vi "Table Manager.vi"(6 "Entry ID in":T1, 8 "Operation":T2, 10 "Entry Name":string) -> (0 "Entries":cluster{"Entry IDs":T1[], "Names":string[]}, 1 "Success":bool, 2 "Entry ID":T1, 4 "Entry Name":string)   [LabVIEW 2017]
doc: "Manges the Name to Entry ID map. Can be used to lookup an entry's ID, add, delete, etc."
uses:
  <vilib>/Rock Robotics/Network Tables/Field ID.ctl
  <vilib>/Rock Robotics/Network Tables/Make Table Operation.ctl
  <vilib>/Rock Robotics/Network Tables/NT Globals.vi
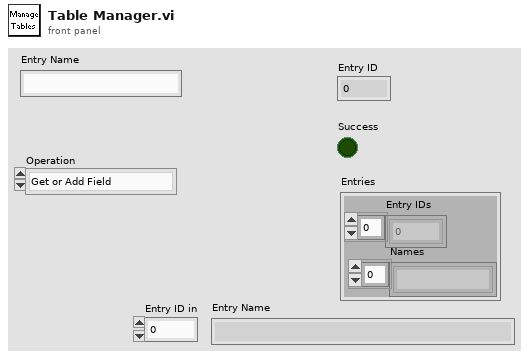
[diagram p1: front panel]
types:
  T1 = typedef "Field ID.ctl" = i32
  T2 = typedef "Make Table Operation.ctl" = enum16{"Get or Add Field", "Get Field or Add Temp", "Replace Temp ID", "Get Field ID - No Add", "Get Table Field IDs", "Get Field ID Info", "Move Field to Temp", "Validate", "Remove Field", "Remove All"}
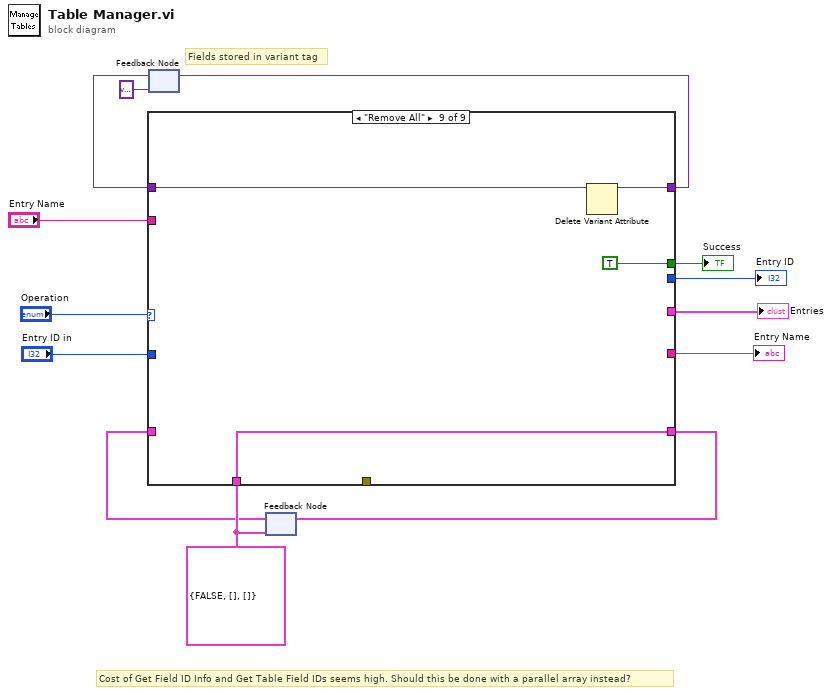
[diagram p0: block diagram]
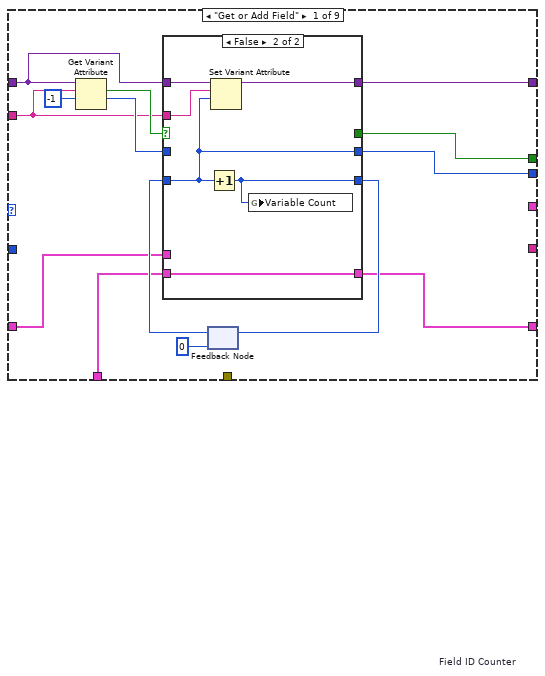
[diagram p2: hidden frame]
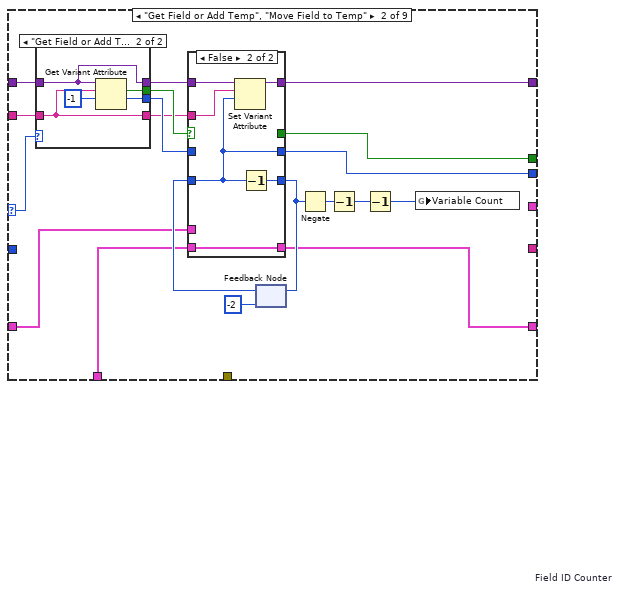
[diagram p4: hidden frame]
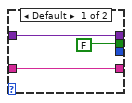
[diagram p5: hidden frame]
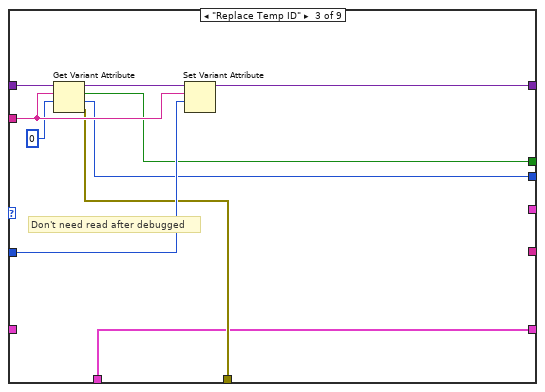
[diagram p7: hidden frame]
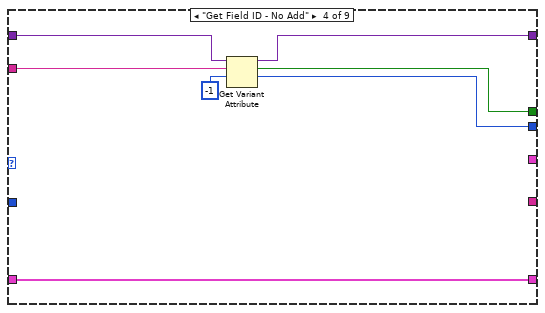
[diagram p8: hidden frame]
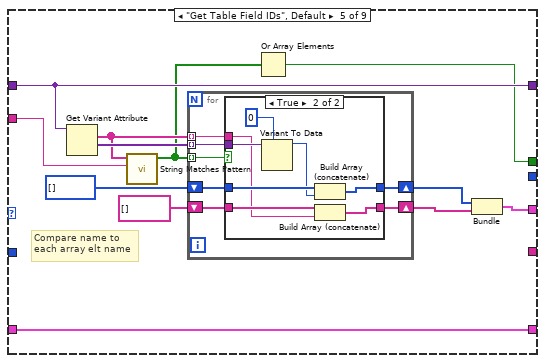
[diagram p9: hidden frame]
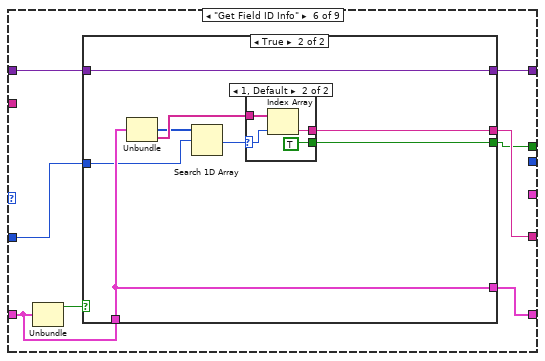
[diagram p11: hidden frame]
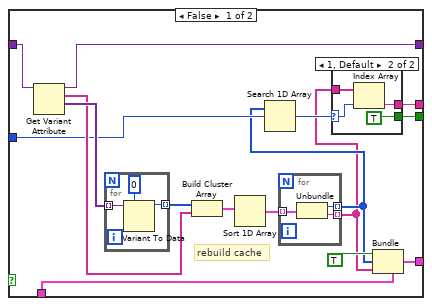
[diagram p12: hidden frame]
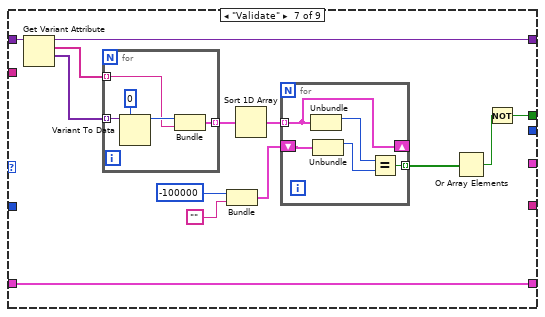
[diagram p15: hidden frame]
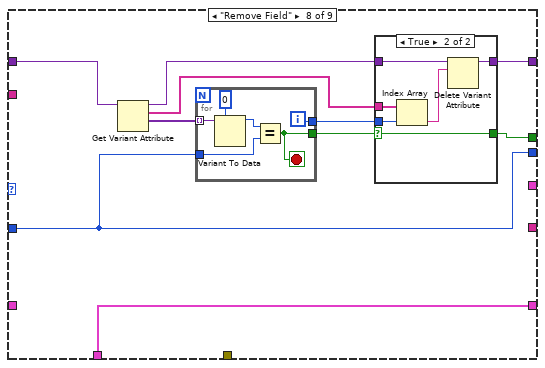
[diagram p16: hidden frame]
diagram:
  w3 = cluster{bool, i32[], string[]} {FALSE, [], []}
  # "Cost of Get Field ID Info and Get Table Field IDs seems high. Should this be done with a parallel array instead?"
  # "Fields stored in variant tag"
  n1 = feedback #1(variant ("Variant")) -> (w7:variant)
  n2 = feedback #2(w3) -> (w2:cluster{bool, i32[], string[]})
  n3 = case shown="\"Remove All\"" "Operation" {
    selector: "Operation" -> [_ w48 _ _ _ _ _ _ _]
    tunnel: w7 -> [w17 w50 w86 w89 w105 w127 w181 w197 w217]
    tunnel: [w21 w51 w81 w88 w105 w126 w180 w194 w219] -> w8
    tunnel: [w25 w55 w82 w91 w95 w124 w171 w196 TRUE] -> w12
    tunnel: "Entry Name" -> [w20 w47 w84 w93 w98 _ _ _ _]
    tunnel: [w26 w56 w79 w92 _ _ _ w193 _] -> w10
    tunnel: "Entry ID in" -> [_ _ w83 _ _ w130 _ w193 _]
    tunnel: [_ _ _ _ _ w125 _ _ _] -> w6
    tunnel: [_ _ _ _ w101 _ _ _ _] -> w4
    tunnel: [_ _ w78 _ _ _ _ _ _] -> _
    tunnel: w3 -> [w15 w40 w77 _ _ _ _ w192 w216]
    tunnel: w2 -> [w16 w41 _ w87 w94 w128 w169 _ _]
    tunnel: [w14 w39 w77 w87 w94 w123 w169 w192 w216] -> w1
    frame "Get or Add Field" {
      n4 = Get Variant Attribute(Variant=w17, name=w20, default value (empty Variant)=-1) -> (found=w24:bool, value=w23:i32)  [unwired: 1 in, 2 out]
      n5 = feedback #3 "Field ID Counter"(0) -> (w19:i32)
      n6 = case shown="False" w24 {
        selector: w24 -> [w30 _]
        tunnel: w17 -> [w32 w37]
        tunnel: [w32 w36] -> w21
        tunnel: w20 -> [_ w38]
        tunnel: [w30 _] -> w25
        tunnel: w19 -> [w29 w35]
        tunnel: [w31 w35] -> w26
        tunnel: w23 -> [w31 _]
        tunnel: [w29 w34] -> w18
        tunnel: w16 -> [w28 _]
        tunnel: w15 -> [_ w33]
        tunnel: [w28 w33] -> w14
        frame True {
          # "Already present"
        }
        frame False {
          n7 = Increment(x=w35) -> (x+1=w34:i32)
          n8 = Set Variant Attribute(Variant=w37, name=w38, value=w35) -> (Variant out=w36:variant)  [unwired: 1 in, 2 out]
          n9 = global write "NT Globals.vi" "Variable Count"(w34) -> ()
        }
      }
      n10 = feedback-in #3(w18) -> ()
    }
    frame "Get Field or Add Temp", "Move Field to Temp" {
      n11 = case shown="\"Get Field or Add Temp\"" w48 {
        tunnel: [FALSE ("Autonomous") w65] -> w54
        tunnel: [_ w64] -> w53
        tunnel: [w59 w61] -> w52
        tunnel: w50 -> [w59 w61]
        tunnel: w47 -> [w60 w63]
        tunnel: [w60 w63] -> w46
        frame Default {
        }
        frame "Get Field or Add Temp" {
          n12 = Get Variant Attribute(Variant=w61, name=w63, default value (empty Variant)=-1) -> (found=w65:bool, value=w64:i32)  [unwired: 1 in, 2 out]
        }
      }
      n13 = feedback #4 "Field ID Counter"(-2) -> (w49:i32)
      n14 = case shown="False" w54 {
        selector: w54 -> [w68 _]
        tunnel: w52 -> [w70 w75]
        tunnel: [w70 w74] -> w51
        tunnel: w46 -> [_ w76]
        tunnel: [w68 _] -> w55
        tunnel: w49 -> [w67 w73]
        tunnel: [w69 w73] -> w56
        tunnel: w53 -> [w69 _]
        tunnel: [w67 w72] -> w45
        tunnel: w41 -> [w66 _]
        tunnel: w40 -> [_ w71]
        tunnel: [w66 w71] -> w39
        frame True {
          # "Already\npresent"
        }
        frame False {
          n15 = Set Variant Attribute(Variant=w75, name=w76, value=w73) -> (Variant out=w74:variant)  [unwired: 1 in, 2 out]
          n16 = Decrement(x=w73) -> (x-1=w72:i32)
        }
      }
      n17 = feedback-in #4(w45) -> ()
      n18 = Negate(x=w45) -> (-x=w44:i32)
      n19 = Decrement(x=w44) -> (x-1=w43:i32)
      n20 = Decrement(x=w43) -> (x-1=w42:i32)
      n21 = global write "NT Globals.vi" "Variable Count"(w42) -> ()
    }
    frame "Replace Temp ID" {
      # "Don't need read after debugged"
      n22 = Get Variant Attribute(Variant=w86, name=w84, default value (empty Variant)=T1 0 ("Entry ID")) -> (duplicate Variant=w85:variant, found=w82:bool, value=w79:T1, error out=w78:errorcluster)  [unwired: 1 in]
      n23 = Set Variant Attribute(Variant=w85, name=w84, value=w83) -> (Variant out=w81:variant)  [unwired: 1 in, 2 out]
    }
    frame "Get Field ID - No Add" {
      n24 = Get Variant Attribute(Variant=w89, name=w93, default value (empty Variant)=-1) -> (duplicate Variant=w88:variant, found=w91:bool, value=w92:i32)  [unwired: 1 in, 1 out]
    }
    frame "Get Table Field IDs", Default {
      # "Compare name to\neach array elt name"
      n25 = Get Variant Attribute(Variant=w105) -> (names=w97:string[], values=w104:variant[])  [unwired: 3 in, 2 out]
      n26 = call <vilib>:"String Matches Pattern.vi"("Pattern"=w98, "Names"=w97) -> ("Matching"=w96:bool[])  [unwired: 9 in]
      n27 = for {
        tunnel: w104 -> [w112] mode=indexing
        tunnel: w97 -> [w107] mode=indexing
        shift-right: [w109] -> w102
        shift-left: i32[] [] -> [w111]
        shift-right: [w108] -> w103
        shift-left: string[] [] ("names") -> [w110]
        tunnel: w96 -> [w106] mode=indexing
        n28 = case shown="True" w106 {
          tunnel: w112 -> [_ w122]
          tunnel: w111 -> [w114 w118]
          tunnel: w110 -> [w113 w120]
          tunnel: [w114 w117] -> w109
          tunnel: [w113 w119] -> w108
          tunnel: w107 -> [_ w115]
          frame False {
          }
          frame True {
            n29 = Variant To Data(type=0, Variant=w122) -> (data=w116:i32)  [unwired: 1 in, 1 out]
            n30 = Build Array (concatenate)(w118, w116) -> (w117:i32[])
            n31 = Build Array (concatenate)(w120, w115) -> (w119:string[])
          }
        }
      }
      n32 = Or Array Elements(Boolean array=w96) -> (logical OR=w95:bool)
      n33 = Bundle(w102, "names"=w103) -> (w101:cluster{i32[], "names":string[]})  [unwired: 1 in]
    }
    frame "Get Field ID Info" {
      n34 = Unbundle(w128) -> (w129:bool)  [unwired: 2 out]
      n35 = case shown="True" w129 {
        tunnel: w130 -> [w134 w159]
        tunnel: [w146 w162] -> w125
        tunnel: w127 -> [w145 w161]
        tunnel: [w144 w161] -> w126
        tunnel: [w143 w163] -> w124
        tunnel: [w141 w160] -> w123
        tunnel: w128 -> [w140 w160]
        frame False {
          # "rebuild cache"
          n36 = Get Variant Attribute(Variant=w145) -> (duplicate Variant=w144:variant, names=w137:string[], values=w139:variant[])  [unwired: 3 in, 1 out]
          n37 = for {
            tunnel: w139 -> [w152] mode=indexing
            tunnel: [w150] -> w138 mode=indexing
            n38 = Variant To Data(type=0, Variant=w152) -> (data=w150:i32)  [unwired: 1 in, 1 out]
          }
          n39 = Build Cluster Array(w138, w137) -> (w136:cluster{i32, string}[])
          n40 = Sort 1D Array(array=w136) -> (sorted array=w135:cluster{i32, string}[])
          n41 = for {
            tunnel: w135 -> [w149] mode=indexing
            tunnel: [w148] -> w133 mode=indexing
            tunnel: [w147] -> w131 mode=indexing
            n42 = Unbundle(w149) -> (w148:i32, w147:string)
          }
          n43 = Search 1D Array(1D array=w133, element=w134) -> (index of element=w132:i32)  [unwired: 1 in]
          n44 = case shown="1, Default" w132 {
            selector: w132 -> [_ w154]
            tunnel: w131 -> [_ w156]
            tunnel: [_ w155] -> w146
            tunnel: [_ TRUE] -> w143
            frame -1 {
            }
            frame 1, Default {
              n45 = Index Array(array=w156, index=w154) -> (element=w155:string)
            }
          }
          n46 = Bundle(cluster=w140, TRUE, w133, w131) -> (w141:cluster{bool, i32[], string[]})
        }
        frame True {
          n47 = Unbundle(w160) -> (w158:i32[], w164:string[])  [unwired: 1 out]
          n48 = Search 1D Array(1D array=w158, element=w159) -> (index of element=w157:i32)  [unwired: 1 in]
          n49 = case shown="1, Default" w157 {
            selector: w157 -> [_ w166]
            tunnel: w164 -> [_ w168]
            tunnel: [_ w167] -> w162
            tunnel: [_ TRUE] -> w163
            frame -1 {
            }
            frame 1, Default {
              n50 = Index Array(array=w168, index=w166) -> (element=w167:string)
            }
          }
        }
      }
    }
    frame "Validate" {
      n51 = Get Variant Attribute(Variant=w181) -> (duplicate Variant=w180:variant, names=w178:string[], values=w179:variant[])  [unwired: 3 in, 1 out]
      n52 = for {
        tunnel: w179 -> [w190] mode=indexing
        tunnel: w178 -> [w188] mode=indexing
        tunnel: [w187] -> w177 mode=indexing
        n53 = Variant To Data(type=0, Variant=w190) -> (data=w189:i32)  [unwired: 1 in, 1 out]
        n54 = Bundle(w189, w188) -> (w187:cluster{i32, string})  [unwired: 1 in]
      }
      n55 = Bundle(-100000, "") -> (w174:cluster{i32, string})  [unwired: 1 in]
      n56 = Sort 1D Array(array=w177) -> (sorted array=w176:cluster{i32, string}[])
      n57 = for {
        shift-right: [w185] -> _
        shift-left: w174 -> [w186]
        tunnel: w176 -> [w185] mode=indexing
        tunnel: [w182] -> w172 mode=indexing
        n58 = Unbundle(w185) -> (w184:i32)  [unwired: 1 out]
        n59 = Unbundle(w186) -> (w183:i32)  [unwired: 1 out]
        n60 = Equal?(x=w184, y=w183) -> (x = y?=w182:bool)
      }
      n61 = Or Array Elements(Boolean array=w172) -> (logical OR=w170:bool)
      n62 = Not(x=w170) -> (.not. x?=w171:bool)
    }
    frame "Remove Field" {
      n63 = Get Variant Attribute(Variant=w197) -> (duplicate Variant=w195:variant, names=w199:string[], values=w201:variant[])  [unwired: 3 in, 1 out]
      n64 = for {
        tunnel: w201 -> [w215] mode=indexing
        tunnel: w193 -> [w212]
        tunnel: [w211] -> w200
        tunnel: [w210] -> w198
        i -> [w210]
        stop <- w211 stop-if-true
        n65 = Variant To Data(type=0, Variant=w215) -> (data=w213:i32)  [unwired: 1 in, 1 out]
        n66 = Equal?(x=w213, y=w212) -> (x = y?=w211:bool)
      }
      n67 = case shown="True" w200 {
        selector: w200 -> [w202 w207]
        tunnel: w199 -> [_ w209]
        tunnel: w198 -> [_ w208]
        tunnel: [w202 w207] -> w196
        tunnel: w195 -> [w203 w205]
        tunnel: [w203 w204] -> w194
        frame False {
        }
        frame True {
          n68 = Index Array(array=w209, index=w208) -> (element=w206:string)
          n69 = Delete Variant Attribute(6:w206, 7:w205) -> (3:w204:variant)  [unwired: 1 in, 2 out]
        }
      }
    }
    frame "Remove All" {
      n70 = Delete Variant Attribute(7:w217) -> (3:w219:variant)  [unwired: 2 in, 2 out]
    }
  }
  "Entry ID" <- w10
  "Success" <- w12
  "Entry Name" <- w6
  "Entries" <- w4
  n71 = feedback-in #1(w8) -> ()
  n72 = feedback-in #2(w1) -> ()
